vi "Get Control Data.vi"(8 "error in (no error)":errorcluster, 11 "VI in":refnum<vi>) -> (0 "error out":errorcluster, 2 "Control Data":T1[](array[typedef]), 3 "VI out":refnum<vi>)   [LabVIEW 2023, in "VI Properties Editor.lvlib"]
doc: "Gets all control data for <B>VI in</B>."
uses:
  VI Properties Editor.lvlib
  CTLs/Control Properties.ctl
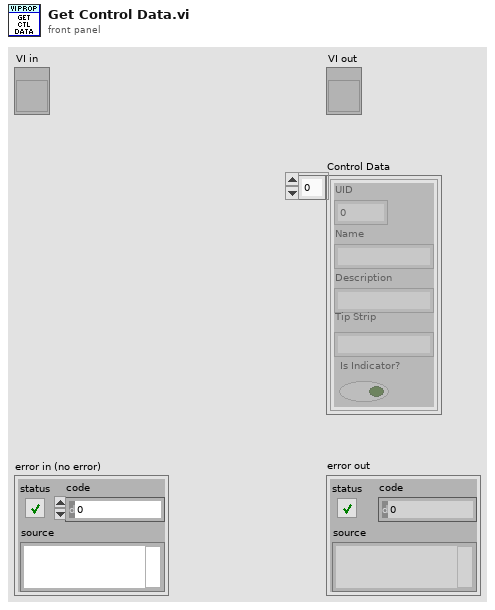
[diagram p1: front panel]
types:
  T1 = typedef "VI Properties Editor.lvlib/Control Properties.ctl" = cluster{"UID":i32, "Name":string, "Description":string, "Tip Strip":string, "Is Indicator?":bool}
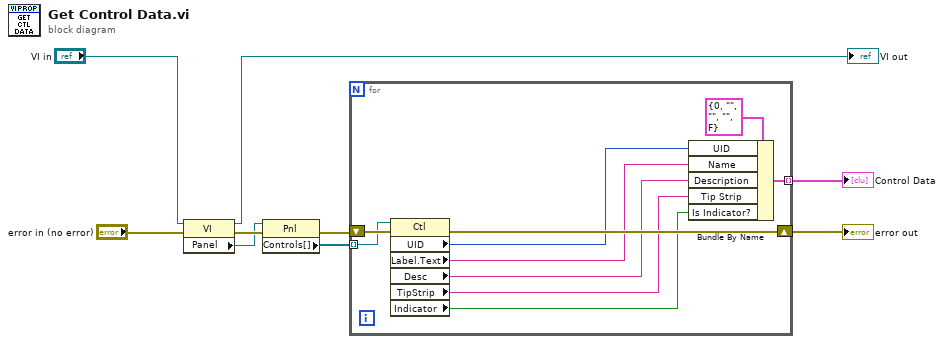
[diagram p0: block diagram]
diagram:
  n1 = property class="VI"(reference="VI in", error in="error in (no error)") -> (reference out=→"VI out":refnum<vi>, error out=w4:errorcluster, "Panel"=w3:refnum<vi>)
  n2 = property class="Pnl"(reference=w3, error in=w4) -> (error out=w9:errorcluster, "Controls[]"=w8:refnum<vi>[])  [unwired: 1 out]
  n3 = for {
    tunnel: w8 -> [w17] mode=indexing
    shift-right: [w18] -> w7
    shift-left: w9 -> [w19]
    tunnel: [w13] -> w5 mode=indexing
    n4 = property class="Ctl"(reference=w17, error in=w19) -> (error out=w18:errorcluster, "UID"=w10:i32, "Label.Text"=w12:string, "Desc"=w15:string, "TipStrip"=w14:string, "Indicator"=w11:bool)  [unwired: 1 out]
    n5 = Bundle By Name(cluster=T1 {"UID"=0, "Name"="", "Description"="", "Tip Strip"="", "Is Indicator?"=FALSE} ("Control Properties"), "UID"=w10, "Name"=w12, "Description"=w15, "Tip Strip"=w14, "Is Indicator?"=w11) -> (w13:T1)
  }
  "error out" <- w7
  "Control Data" <- w5
